vi "MenuHandler.vi"(5 "tree control":refnum<vi>, 7 "main queue":refnum<queue>, 8 "error in":errorcluster, 9 "parameters":variant, 10 "menu string":string, 11 "Digitizer Instrument in":refnum<class "Digitizer Instrument.lvclass">) -> (0 "error out":errorcluster, 1 "refresh tree?":bool, 2 "Unhandled":bool, 3 "Digitizer Instrument out":refnum<class "Digitizer Instrument.lvclass">)   [LabVIEW 2025, in "Digitizer.lvlib" / "Digitizer Instrument.lvclass"]
doc: "Copyright 2017 National Instruments Corporation\n\nLicensed under the Apache License, Version 2.0 (the \"License\"); you may not use this file except in compliance with the License. You may obtain a copy of the License at http://www.apache.org/licenses/LICENSE-2.0\nUnless required by applicable law or agreed to in writing, software distributed under the License is distributed on an \"AS IS\" BASIS, WITHOUT WARRANTIES OR CONDITIONS OF ANY KIND, either express or implied. See the License for the specific language governing permissions and limitations under the License."
uses:
  Digitizer Instrument.lvclass
  Users/Public/Documents/Sandia National Labs/TSS Plugin/Abstract Engine.lvlibp/Abstract Instrument/Abstract Instrument.lvclass
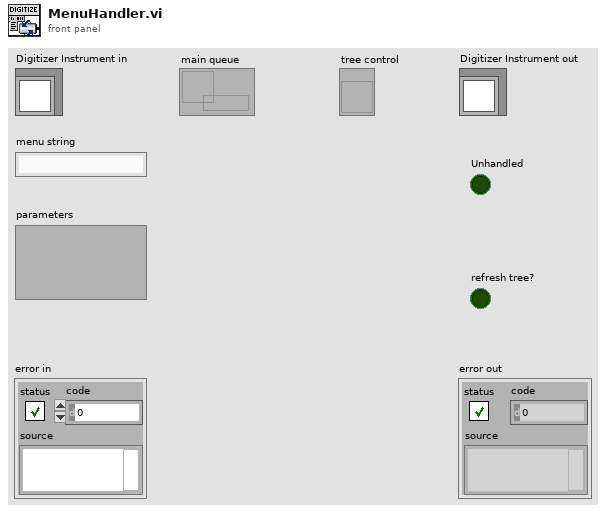
[diagram p1: front panel]
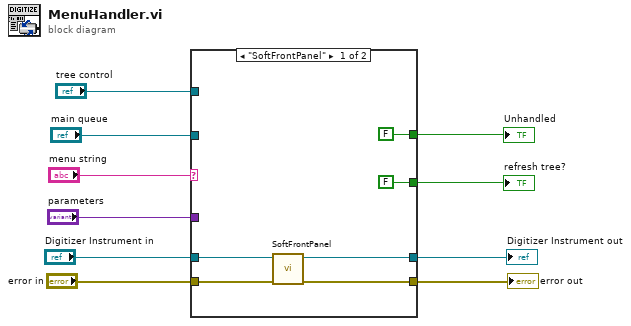
[diagram p0: block diagram]
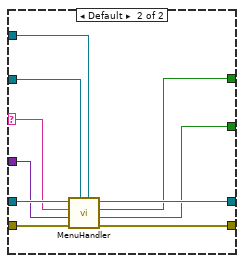
[diagram p2: hidden frame]
diagram:
  n1 = case shown="\"SoftFrontPanel\"" "menu string" {
    selector: "menu string" -> [_ w22]
    tunnel: "error in" -> [w12 w26]
    tunnel: [w11 w25] -> w8
    tunnel: "Digitizer Instrument in" -> [w14 w24]
    tunnel: [w13 w23] -> w6
    tunnel: "parameters" -> [_ w21]
    tunnel: "main queue" -> [_ w20]
    tunnel: "tree control" -> [_ w19]
    tunnel: [FALSE ("Unhandled") w18] -> w2
    tunnel: [FALSE ("refresh tree?") w17] -> w1
    frame "SoftFrontPanel" {
      n2 = call "SoftFrontPanel.vi"("error in (no error)"=w12, "Digitizer Instrument"=w14) -> ("error out"=w11:errorcluster, "Digitizer Instrument out"=w13:refnum<class "Digitizer Instrument.lvclass">)  [unwired: 8 in]
    }
    frame Default {
      n3 = call-parent "MenuHandler.vi"("tree control"=w19, "main queue"=w20, "error in"=w26, "parameters"=w21, "menu string"=w22, "CEF_serializable node in"=w24) -> ("error out"=w25:errorcluster, "refresh tree?"=w17:bool, "Unhandled"=w18:bool, "CEF_serializable node out"=w23:refnum<class "Digitizer Instrument.lvclass">)  [unwired: 2 in]
    }
  }
  "error out" <- w8
  "Digitizer Instrument out" <- w6
  "Unhandled" <- w2
  "refresh tree?" <- w1
